vi "register for events.vi"(8 "error in":errorcluster, 11 "websocket standalone server in":refnum<class "websocket standalone server.lvclass">) -> (0 "error out":errorcluster, 3 "event registration":refnum<event-registration>)   [LabVIEW 2016, in "websocket standalone server.lvclass"]
uses:
  websocket standalone server.lvclass
  websocket data packet.ctl
  websocket message type.ctl
  websocket sourced packet.ctl
  websocket standalone server.lvclass/websocket standalone server.ctl
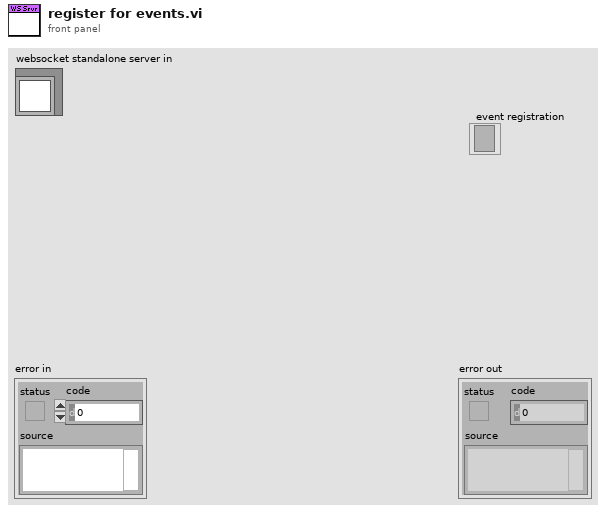
[diagram p1: front panel]
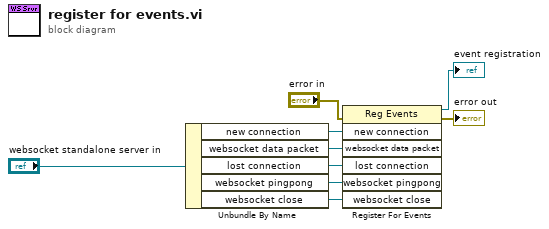
[diagram p0: block diagram]
diagram:
  n1 = Unbundle By Name("websocket standalone server in") -> ("new connection"=w6:refnum<user-event>, "websocket data packet"=w2:refnum<user-event>, "lost connection"=w3:refnum<user-event>, "websocket pingpong"=w4:refnum<user-event>, "websocket close"=w5:refnum<user-event>)
  n2 = register-events(error in="error in", w6, w2, w3, w4, w5) -> (reference out=→"event registration":refnum<event-registration>, error out=→"error out":errorcluster)  [unwired: 1 in]
